vi "RTS Get CMD Data Volt Freq.vi"(8 "Error In":errorcluster, 10 "Data String":string) -> (0 "Error Out":errorcluster, 1 "Voltage":dbl, 2 "Frequency":T1 items=["60 Hz", "50 Hz"], 3 "Wh Reset 2":T2 caption="Wh Reset")   [LabVIEW 2016]
uses:
  Type Definitions/RTS Reset Watt Hours.ctl
  Type Definitions/RTS Frequency Selector.ctl
  Type Definitions/RTS Custom Commands.ctl
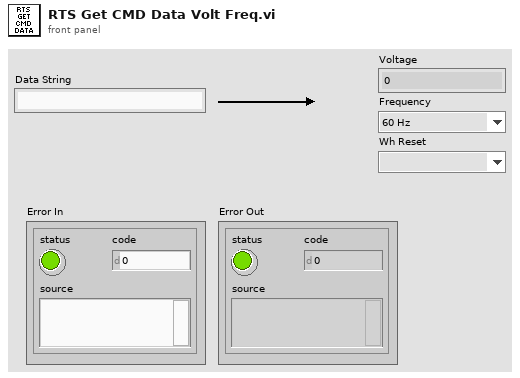
[diagram p1: front panel]
types:
  T1 = typedef "RTS Frequency Selector.ctl" = u16
  T2 = typedef "RTS Reset Watt Hours.ctl" = enum16{"", "Reset Watt Hours"}
  T3 = typedef "RTS Custom Commands.ctl" = string
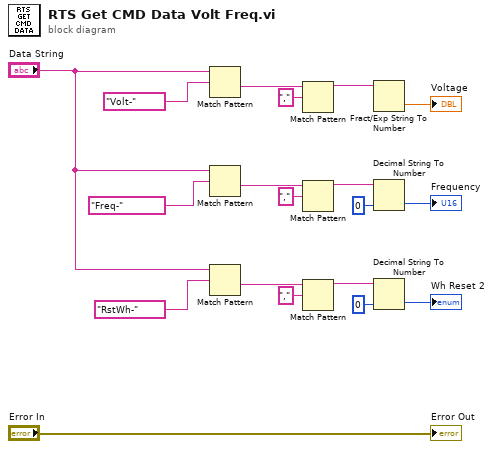
[diagram p0: block diagram]
diagram:
  n1 = Match Pattern(string="Data String", regular expression=T3 "Volt-" ("Custom CMD")) -> (after substring=w18:string)  [unwired: 1 in, 3 out]
  n2 = Match Pattern(string="Data String", regular expression=T3 "Freq-" ("Custom CMD 2")) -> (after substring=w13:string)  [unwired: 1 in, 3 out]
  n3 = Match Pattern(string="Data String", regular expression=T3 "RstWh-" ("Custom CMD 3")) -> (after substring=w8:string)  [unwired: 1 in, 3 out]
  n4 = Match Pattern(string=w18, regular expression=",") -> (before substring=w16:string)  [unwired: 1 in, 3 out]
  n5 = Match Pattern(string=w13, regular expression=",") -> (before substring=w10:string)  [unwired: 1 in, 3 out]
  n6 = Match Pattern(string=w8, regular expression=",") -> (before substring=w3:string)  [unwired: 1 in, 3 out]
  n7 = Fract/Exp String To Number(string=w16) -> (number=→"Voltage":dbl)  [unwired: 3 in, 1 out]
  n8 = Decimal String To Number(string=w10, default (0L)=u16 0 ("default (0 I32)")) -> (number=→"Frequency":u16)  [unwired: 1 in, 1 out]
  n9 = Decimal String To Number(string=w3, default (0L)=u16 0 ("default (0 I32)")) -> (number=→"Wh Reset 2":u16)  [unwired: 1 in, 1 out]
  "Error Out" <- "Error In"
